vi "Cycle Period FGV.vi"(7 "Write":bool, 8 "error in (no error)":errorcluster, 11 "Cycle Period In (ms)":dbl) -> (0 "error out":errorcluster, 3 "Cycle Period Out (ms)":dbl)   [LabVIEW 2018]
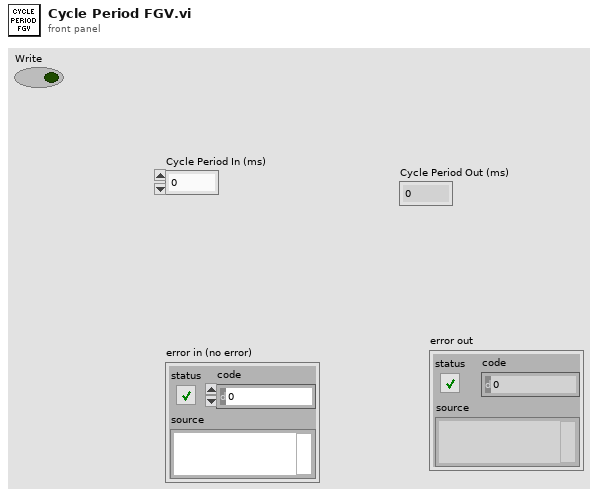
[diagram p1: front panel]
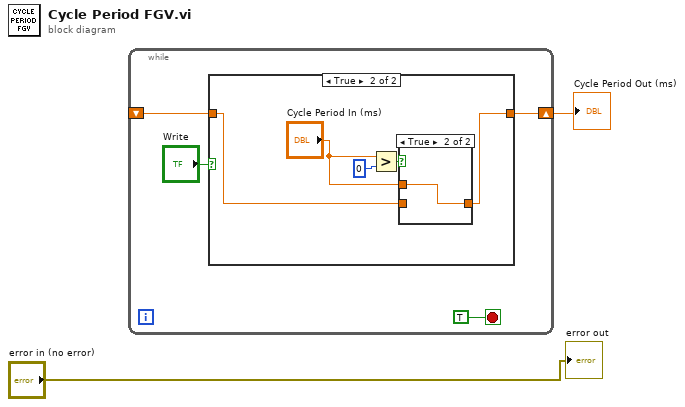
[diagram p0: block diagram]
diagram:
  n1 = while {
    shift-right: [w4] -> w2
    shift-left: _ -> [w3]
    stop <- TRUE stop-if-true
    n2 = case shown="True" "Write" {
      tunnel: [w7 w10] -> w4
      tunnel: w3 -> [w7 w8]
      frame False {
      }
      frame True {
        n3 = Greater?(x="Cycle Period In (ms)", y=0) -> (0:w11:bool)
        n4 = case shown="True" w11 {
          tunnel: "Cycle Period In (ms)" -> [_ w14]
          tunnel: [w13 w14] -> w10
          tunnel: w8 -> [w13 _]
          frame False {
          }
          frame True {
          }
        }
      }
    }
  }
  "Cycle Period Out (ms)" <- w2
  "error out" <- "error in (no error)"
